vi "Render Comment.vi"(8 "Error In":errorcluster, 10 "Comment":refnum<class "Comment.lvclass">, 11 "Context In":refnum<class "Context.lvclass">) -> (0 "Error Out":errorcluster, 2 "Output":string, 3 "Context Out":refnum<class "Context.lvclass">)   [LabVIEW 2018, in "Toolkit.lvlib"]
uses:
  Toolkit.lvlib
  Context/Context/Context.lvclass
  Nodes/Comment/Comment.lvclass
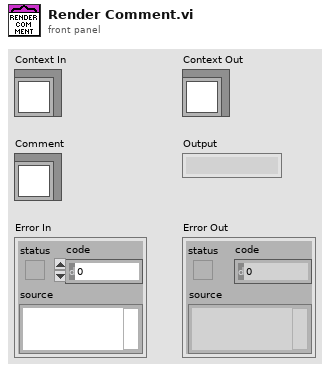
[diagram p1: front panel]
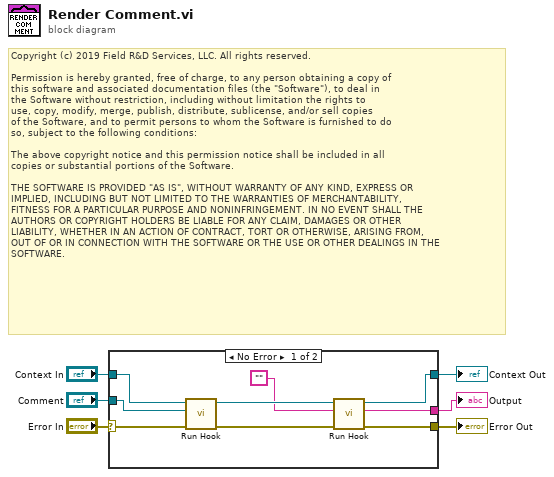
[diagram p0: block diagram]
diagram:
  # "Copyright (c) 2019 Field R&D Services, LLC. All rights reserved.\n\nPermission is hereby granted, free of charge, to any person obtaining a copy of\nthis software and associated documentation files (the \"Software\"), to deal in\nthe Software without restriction, including without limitation the rights to\nuse, copy, modify, merge, publish, distribute, sublicense, and/or sell copies\nof the Software, and to permit persons to whom the Software is furnished to do\nso, subject to the following conditions:\n\nThe above copyright notice and this permission notice shall be included in all\ncopies or substantial portions of the Software.\n\nTHE SOFTWARE IS PROVIDED \"AS IS\", WITHOUT WARRANTY OF ANY KIND, EXPRESS OR\nIMPLIED, INCLUDING BUT NOT LIMITED TO THE WARRANTIES OF MERCHANTABILITY,\nFITNESS FOR A PARTICULAR PURPOSE AND NONINFRINGEMENT. IN NO EVENT SHALL THE\nAUTHORS OR COPYRIGHT HOLDERS BE LIABLE FOR ANY CLAIM, DAMAGES OR OTHER\nLIABILITY, WHETHER IN AN ACTION OF CONTRACT, TORT OR OTHERWISE, ARISING FROM,\nOUT OF OR IN CONNECTION WITH THE SOFTWARE OR THE USE OR OTHER DEALINGS IN THE\nSOFTWARE."
  n1 = case shown="No Error" "Error In" {
    selector: "Error In" -> [w10 w17]
    tunnel: [w13 w17] -> w5
    tunnel: "Context In" -> [w11 w16]
    tunnel: [w7 _] -> w3
    tunnel: "Comment" -> [w9 _]
    tunnel: [w12 w16] -> w1
    frame No Error {
      n2 = call-poly "Run Hook.vi"("Error In"=w10, "Comment In"=w9, "Context In"=w11) -> ("Error Out"=w14:errorcluster, "Context Out"=w15:refnum<class "Context.lvclass">)  [unwired: 6 in, 1 out]
      n3 = call-poly "Run Hook.vi"("Error In"=w14, "Output In"="", "Context In"=w15) -> ("Error Out"=w13:errorcluster, "Output Out"=w7:string, "Context Out"=w12:refnum<class "Context.lvclass">)  [unwired: 6 in]
    }
    frame Error {
    }
  }
  "Error Out" <- w5
  "Output" <- w3
  "Context Out" <- w1
